vi "Set Strings from Ref.vi"(8 "error in (no error)":errorcluster, 9 "Language Index (0)":i32, 10 "GObj Refnum":refnum<vi>, 11 "DecorationText in":refnum<class "DecorationText.lvclass">) -> (0 "error out":errorcluster, 3 "DecorationText out":refnum<class "DecorationText.lvclass">)   [LabVIEW 2013, in "SET Project Data.lvlib" / "DecorationText.lvclass"]
uses:
  DecorationText.lvclass
  GObject/GObject.lvclass
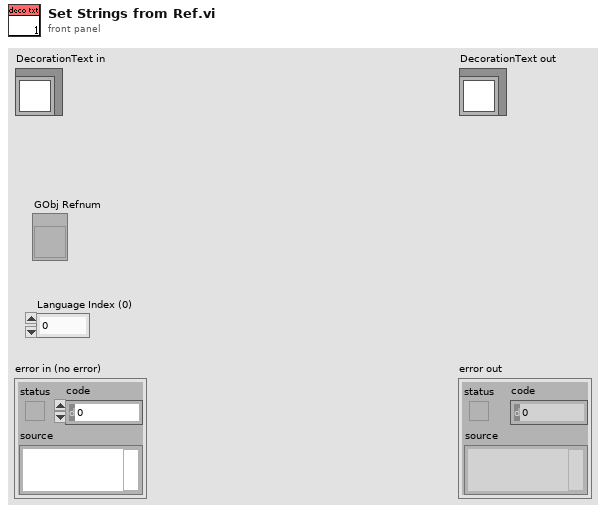
[diagram p1: front panel]
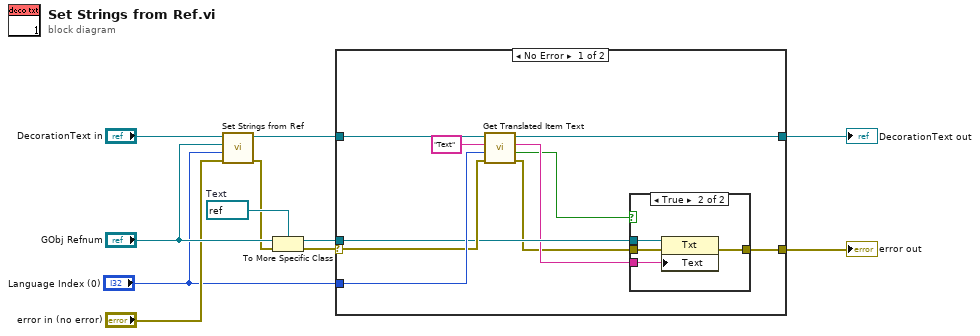
[diagram p0: block diagram]
diagram:
  w11 = refnum<vi> refnum  # Text
  n1 = call-parent "Set Strings from Ref.vi"("error in (no error)"="error in (no error)", "Language Index (0)"="Language Index (0)", "GObj Refnum"="GObj Refnum", "GObject in"="DecorationText in") -> ("error out"=w5:errorcluster, "GObject out"=w7:refnum<class "DecorationText.lvclass">)  [unwired: 6 in]
  n2 = To More Specific Class(target class=w11, reference="GObj Refnum", error in=w5) -> (specific class reference=w9:refnum<vi>, error out=w10:errorcluster)
  n3 = case shown="No Error" w10 {
    selector: w10 -> [w17 w27]
    tunnel: w9 -> [w16 _]
    tunnel: "Language Index (0)" -> [w18 _]
    tunnel: w7 -> [w21 w28]
    tunnel: [w20 w28] -> w2
    tunnel: [w13 w27] -> w1
    frame No Error {
      n4 = call "Get Translated Item Text.vi"("error in (no error)"=w17, "LangIndex (0)"=w18, "ItemName"="Text" ("name"), "GObject in"=w21) -> ("error out"=w14:errorcluster, "Found?"=w12:bool, "Translated Text (ASCII)"=w15:string, "GObject out"=w20:refnum<class "DecorationText.lvclass">)  [unwired: 4 in]
      n5 = case shown="True" w12 {
        tunnel: w16 -> [_ w26]
        tunnel: w15 -> [_ w25]
        tunnel: w14 -> [w22 w24]
        tunnel: [w22 w23] -> w13
        frame False {
        }
        frame True {
          n6 = property class="Txt"(reference=w26, error in=w24, "Text"=w25) -> (error out=w23:errorcluster)  [unwired: 1 out]
        }
      }
    }
    frame Error {
    }
  }
  "error out" <- w1
  "DecorationText out" <- w2
